vi "medidorIXV.vi"(4 "nMedicoes":i16) -> (7 "Tensao Atual":dbl, 8 "Corrente Atual":dbl, 10 "vetorCorrente":dbl[](array[numeric]) format="%#.6g")   [LabVIEW 2012]
panel:
  out "somaCorrente":dbl
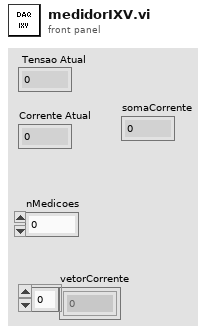
[diagram p1: front panel]
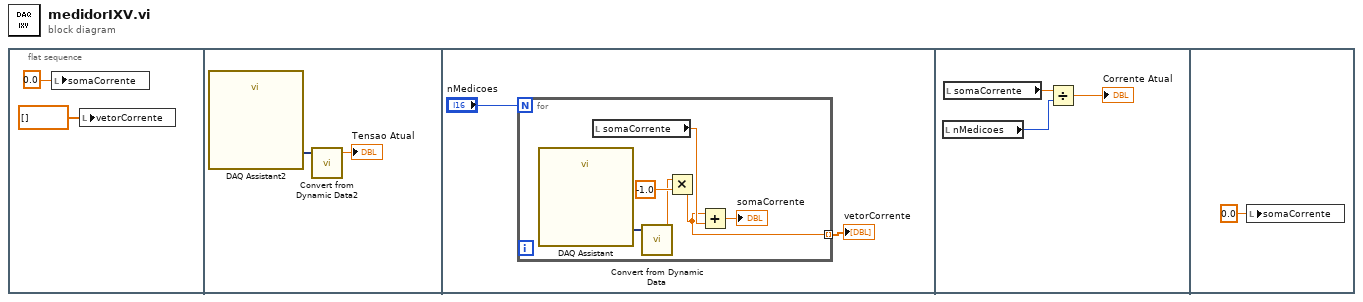
[diagram p0: block diagram]
diagram:
  n1 = flat-sequence {
    frame #0 {
      n2 = local write "somaCorrente"(0.0 ("somaCorrente")) -> ()
      n3 = local write "vetorCorrente"(dbl[] [] ("vetorCorrente")) -> ()
    }
    frame #1 {
      n4 = call "DAQ Assistant2"() -> ("data"=w4:dynamicdata)  [unwired: 17 in, 2 out]
      n5 = call "Convert from Dynamic Data2"("Dynamic Data Type"=w4) -> ("Scalar"=→"Tensao Atual":dbl)  [unwired: 3 in]
    }
    frame #2 {
      n6 = for {
        N: "nMedicoes" -> [_]
        tunnel: [w7] -> w5 mode=indexing
        n7 = call "DAQ Assistant"() -> ("data"=w12:dynamicdata)  [unwired: 17 in, 2 out]
        n8 = local read "somaCorrente"() -> (w11:dbl)
        n9 = call "Convert from Dynamic Data"("Dynamic Data Type"=w12) -> ("Scalar"=w8:dbl)  [unwired: 3 in]
        n10 = Multiply(x=w8, y=-1.0) -> (x*y=w7:dbl)
        n11 = Add(x=w7, y=w11) -> (x+y=→"somaCorrente":dbl)
      }
      "vetorCorrente" <- w5
    }
    frame #3 {
      n12 = local read "nMedicoes"() -> (w15:i16)
      n13 = local read "somaCorrente"() -> (w14:dbl)
      n14 = Divide(x=w14, y=w15) -> (x/y=→"Corrente Atual":dbl)
    }
    frame #4 {
      n15 = local write "somaCorrente"(0.0 ("somaCorrente")) -> ()
    }
  }
